vi "CalculateMieAtSpecificRefractiveIndex.vi"(3 "output control":T3, 4 "data":T4, 5 "X":dbl[](array[numeric]), 6 "a":dbl[](array[numeric])) -> (0 "error out":errorcluster, 1 "f'(X,a)":dbl[][](array[numeric]), 2 "f(X,a)":dbl[](array[numeric]))   [LabVIEW 2013]
doc: "This template is the starting point for creating a model function to be passed to the Nonlinear Curve Fit.vi."
uses:
  <vilib>/gmath/NumericalOptimization/objective function data.ctl
  <vilib>/gmath/NumericalOptimization/LM_output select.ctl
  BaesDataTypeDefinition.ctl
  <vilib>/gmath/NI_Gmath.lvlib
panel:
  out "Enum":T1(ring)
  in  "Extinction ExtinctionUncertainity Size parameter and Number ofS sizes 2":T2={"Extinction"=[], "Extinction Uncertainty"=[], "Size parameters"=[], "Number ofSizes"=0.0, "GeometricCrossSection"=[], "Wave Length"=0.0, "SMPS Sizes"=[], "Concentration"=[], "Double Charge Correction"=FALSE, "Extincation Factor"=1.0, "Diameter Factor"=1.0, "Diameter Offset"=0.0, "Extinction Factor Flag"=FALSE, "Diameter Factor Flag"=FALSE, "Diameter Offset Flag"=FALSE, "Sizes"=[], "ExtinctionOrAbsorptionOrScattering"=0, "Convergence Strength"=enum."Weak"} {"ExtinctionOrAbsorptionOrScattering" scale=0.0..2.0}
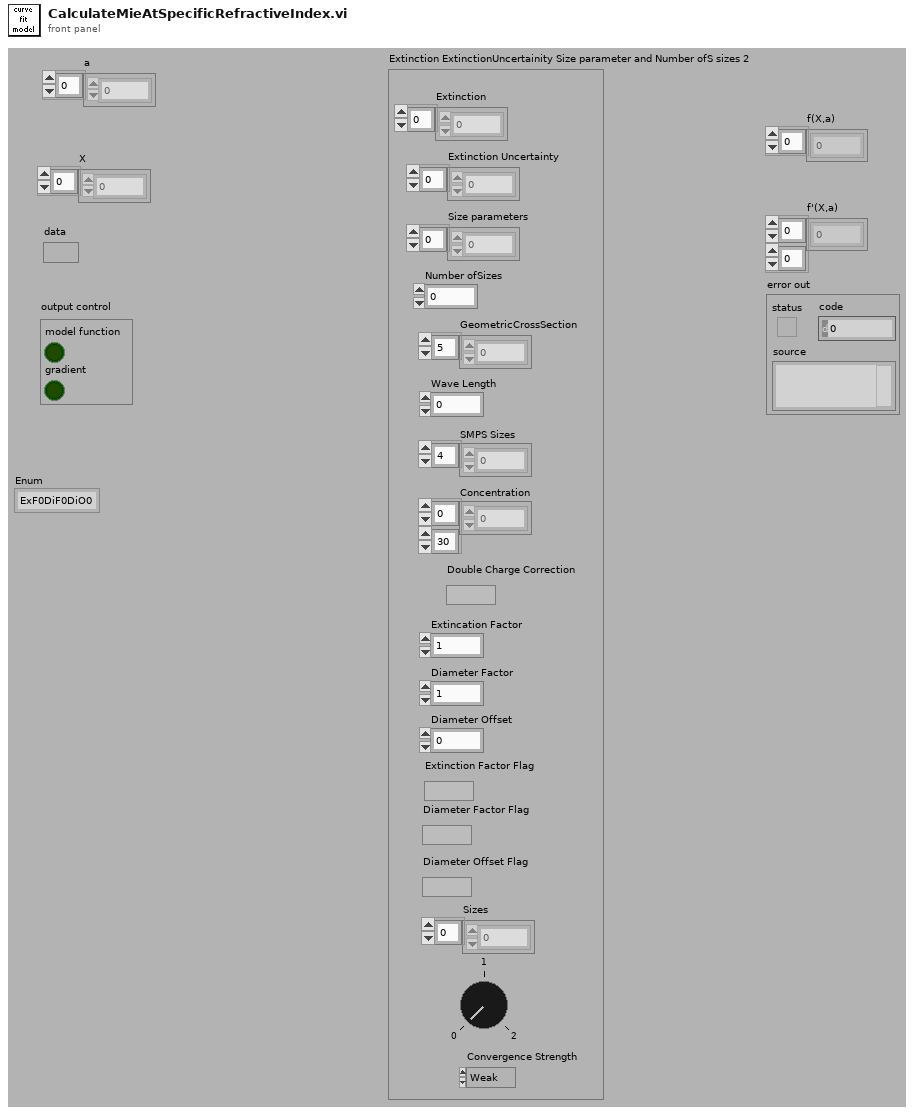
[diagram p1: front panel]
types:
  T1 = enum16{"ExF0DiF0DiO0", "ExF0DiF0DiO1", "ExF0DiF1DiO0", "NotDefined1", "ExF1DiF0DiO0", "ExF1DiF0DiO1", "ExF1DiF1DiO0", "NotDefined"}
  T2 = typedef "BaesDataTypeDefinition.ctl" = cluster{"Extinction":dbl[], "Extinction Uncertainty":dbl[], "Size parameters":dbl[], "Number ofSizes":dbl, "GeometricCrossSection":dbl[], "Wave Length":dbl, "SMPS Sizes":dbl[], "Concentration":dbl[][], "Double Charge Correction":bool, "Extincation Factor":dbl, "Diameter Factor":dbl, "Diameter Offset":dbl, "Extinction Factor Flag":bool, "Diameter Factor Flag":bool, "Diameter Offset Flag":bool, "Sizes":dbl[], "ExtinctionOrAbsorptionOrScattering":i8, "Convergence Strength":enum16{"Weak", "Medium", "Strong"}}
  T3 = typedef "NI_Gmath.lvlib/LM_output select.ctl" = cluster{"model function":bool, "gradient":bool}
  T4 = typedef "NI_Gmath.lvlib/objective function data.ctl" = variant
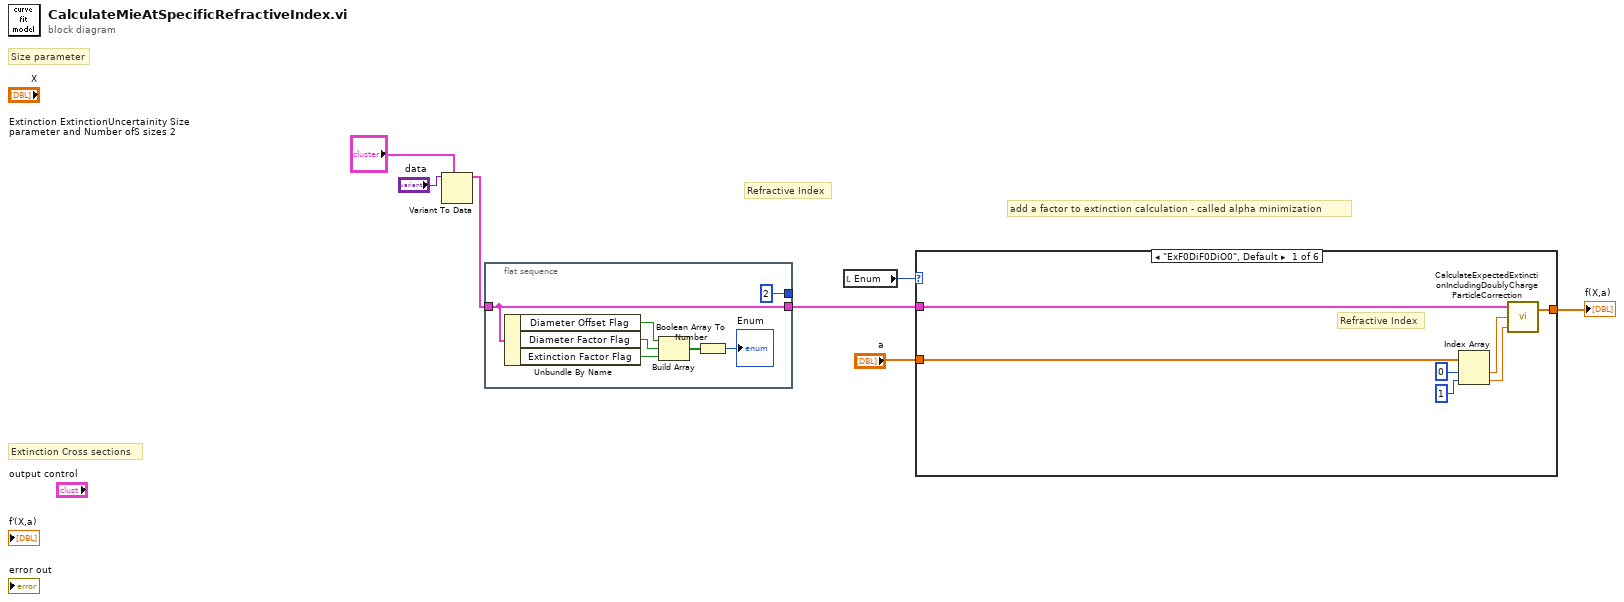
[diagram p0: block diagram]
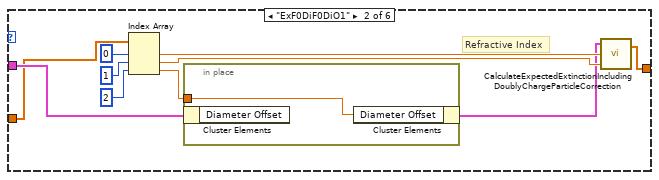
[diagram p2: hidden frame]
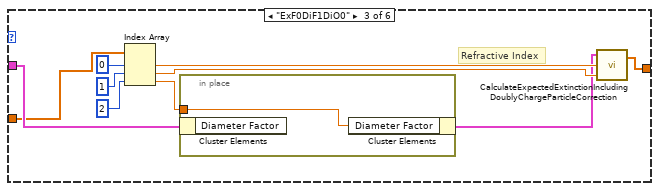
[diagram p3: hidden frame]
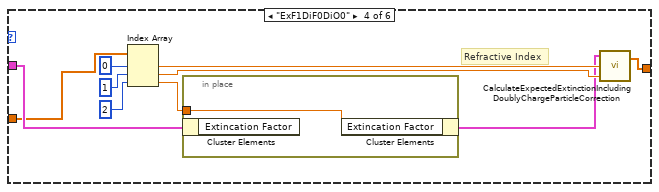
[diagram p4: hidden frame]
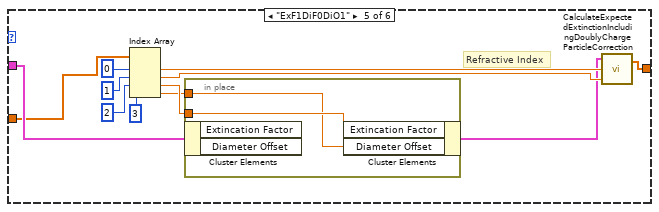
[diagram p5: hidden frame]
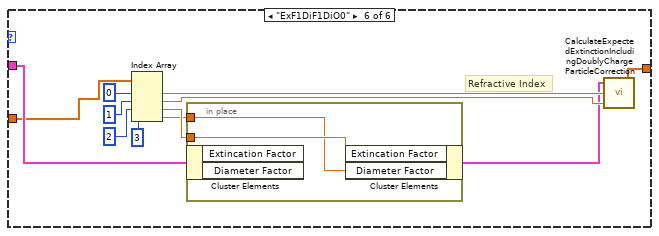
[diagram p6: hidden frame]
diagram:
  # "add a factor to extinction calculation - called alpha minimization"
  # "Extinction Cross sections"
  # "Refractive Index"
  # "Size parameter"
  n1 = Variant To Data(type="Extinction ExtinctionUncertainity Size parameter and Number ofS sizes 2", Variant="data") -> (data=w5:T2)  [unwired: 1 in, 1 out]
  n2 = flat-sequence {
    tunnel: [2 ("index")] -> _
    tunnel: w5 -> [w8]
    tunnel: [w8] -> w2
    frame #0 {
      n3 = Unbundle By Name(w8) -> ("Diameter Offset Flag"=w13:bool, "Diameter Factor Flag"=w12:bool, "Extinction Factor Flag"=w11:bool)
      n4 = Build Array(w13, w12, w11) -> (w10:bool[])
      n5 = Boolean Array To Number(Boolean array=w10) -> (number=→"Enum":u32)
    }
  }
  n6 = local read "Enum"() -> (w3:T1)
  n7 = case shown="\"ExF0DiF0DiO0\", Default" w3 {
    tunnel: w2 -> [w17 w27 w35 w45 w59 w71]
    tunnel: [w16 w23 w34 w46 w56 w70] -> w4
    tunnel: "a" -> [w15 w22 w33 w44 w55 w69]
    frame "ExF0DiF0DiO0", Default {
      # "Refractive Index"
      n8 = Index Array(array=w15, index #1=0 ("index"), index #2=1 ("index")) -> (element #1=w19:dbl, element #2=w18:dbl)
      n9 = call "CalculateExpectedExtinctionIncludingDoublyChargeParticleCorrection.vi"("refractive index, imaginary"=w18, "refractive index, real"=w19, "Extinction ExtinctionUncertainity Size parameter and Number ofS sizes"=w17) -> ("Expected Extinction Cross Section"=w16:sgl[])  [unwired: 1 out]
    }
    frame "ExF0DiF0DiO1" {
      # "Refractive Index"
      n10 = Index Array(array=w22, index #1=0 ("index"), index #2=1 ("index"), index #3=2 ("index")) -> (element #1=w29:dbl, element #2=w28:dbl, element #3=w25:dbl)
      n11 = in-place {
        in-place-border: w25 -> [w32]
        n12 = in-place-cluster #1(w27) -> ()  [unwired: 1 out]
        n13 = in-place-cluster #1("Diameter Offset"=w32) -> (w24:T2)
      }
      n14 = call "CalculateExpectedExtinctionIncludingDoublyChargeParticleCorrection.vi"("refractive index, imaginary"=w28, "refractive index, real"=w29, "Extinction ExtinctionUncertainity Size parameter and Number ofS sizes"=w24) -> ("Expected Extinction Cross Section"=w23:sgl[])  [unwired: 1 out]
    }
    frame "ExF0DiF1DiO0" {
      # "Refractive Index"
      n15 = Index Array(array=w33, index #1=0 ("index"), index #2=1 ("index"), index #3=2 ("index")) -> (element #1=w40:dbl, element #2=w39:dbl, element #3=w37:dbl)
      n16 = in-place {
        in-place-border: w37 -> [w43]
        n17 = in-place-cluster #2(w35) -> ()  [unwired: 1 out]
        n18 = in-place-cluster #2("Diameter Factor"=w43) -> (w36:T2)
      }
      n19 = call "CalculateExpectedExtinctionIncludingDoublyChargeParticleCorrection.vi"("refractive index, imaginary"=w39, "refractive index, real"=w40, "Extinction ExtinctionUncertainity Size parameter and Number ofS sizes"=w36) -> ("Expected Extinction Cross Section"=w34:sgl[])  [unwired: 1 out]
    }
    frame "ExF1DiF0DiO0" {
      # "Refractive Index"
      n20 = Index Array(array=w44, index #1=0 ("index"), index #2=1 ("index"), index #3=2 ("index")) -> (element #1=w51:dbl, element #2=w50:dbl, element #3=w48:dbl)
      n21 = in-place {
        in-place-border: w48 -> [w54]
        n22 = in-place-cluster #3(w45) -> ()  [unwired: 1 out]
        n23 = in-place-cluster #3("Extincation Factor"=w54) -> (w47:T2)
      }
      n24 = call "CalculateExpectedExtinctionIncludingDoublyChargeParticleCorrection.vi"("refractive index, imaginary"=w50, "refractive index, real"=w51, "Extinction ExtinctionUncertainity Size parameter and Number ofS sizes"=w47) -> ("Expected Extinction Cross Section"=w46:sgl[])  [unwired: 1 out]
    }
    frame "ExF1DiF0DiO1" {
      # "Refractive Index"
      n25 = Index Array(array=w55, index #1=0 ("index"), index #2=1 ("index"), index #3=2 ("index"), index #4=3 ("index")) -> (element #1=w64:dbl, element #2=w63:dbl, element #3=w61:dbl, element #4=w57:dbl)
      n26 = in-place {
        in-place-border: w61 -> [w68]
        in-place-border: w57 -> [w67]
        n27 = in-place-cluster #4(w59) -> ()  [unwired: 2 out]
        n28 = in-place-cluster #4("Extincation Factor"=w68, "Diameter Offset"=w67) -> (w60:T2)
      }
      n29 = call "CalculateExpectedExtinctionIncludingDoublyChargeParticleCorrection.vi"("refractive index, imaginary"=w63, "refractive index, real"=w64, "Extinction ExtinctionUncertainity Size parameter and Number ofS sizes"=w60) -> ("Expected Extinction Cross Section"=w56:sgl[])  [unwired: 1 out]
    }
    frame "ExF1DiF1DiO0" {
      # "Refractive Index"
      n30 = Index Array(array=w69, index #1=0 ("index"), index #2=1 ("index"), index #3=2 ("index"), index #4=3 ("index")) -> (element #1=w78:dbl, element #2=w77:dbl, element #3=w75:dbl, element #4=w72:dbl)
      n31 = in-place {
        in-place-border: w75 -> [w82]
        in-place-border: w72 -> [w81]
        n32 = in-place-cluster #5(w71) -> ()  [unwired: 2 out]
        n33 = in-place-cluster #5("Extincation Factor"=w82, "Diameter Factor"=w81) -> (w74:T2)
      }
      n34 = call "CalculateExpectedExtinctionIncludingDoublyChargeParticleCorrection.vi"("refractive index, imaginary"=w77, "refractive index, real"=w78, "Extinction ExtinctionUncertainity Size parameter and Number ofS sizes"=w74) -> ("Expected Extinction Cross Section"=w70:sgl[])  [unwired: 1 out]
    }
  }
  "f(X,a)" <- w4
